vi "FlatToRichniswitch_grpc_InitRequest.vi"(5 "OutputClusterType":T1, 11 "InputCluster":T3) -> (3 "OutputCluster":T1)   [LabVIEW 2021, in "NI Switch_client.lvlib"]
uses:
  NI Switch_client.lvlib
  niswitch_grpc_InitRequest_Flat.ctl
  nidevice_grpc_SessionInitializationBehavior.ctl
  niswitch_grpc_InitRequest.ctl
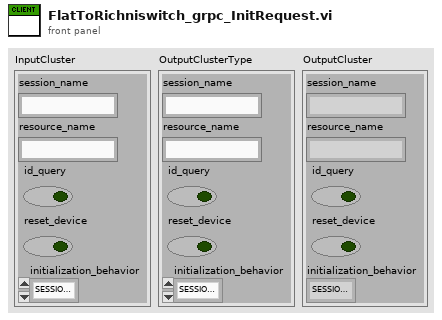
[diagram p1: front panel]
types:
  T1 = typedef "NI Switch_client.lvlib/niswitch_grpc_InitRequest.ctl" = cluster{"session_name":string, "resource_name":string, "id_query":bool, "reset_device":bool, "initialization_behavior":T2}
  T2 = typedef "NI Switch_client.lvlib/nidevice_grpc_SessionInitializationBehavior.ctl" = enum32{"SESSION_INITIALIZATION_BEHAVIOR_UNSPECIFIED", "SESSION_INITIALIZATION_BEHAVIOR_INITIALIZE_NEW", "SESSION_INITIALIZATION_BEHAVIOR_ATTACH_TO_EXISTING"}
  T3 = typedef "NI Switch_client.lvlib/niswitch_grpc_InitRequest_Flat.ctl" = cluster{"session_name":string, "resource_name":string, "id_query":bool, "reset_device":bool, "initialization_behavior":T2}
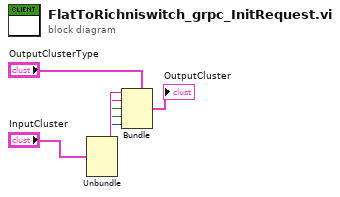
[diagram p0: block diagram]
diagram:
  n1 = Unbundle "Unbundle"("InputCluster") -> ("session_name"=w5:string, "resource_name"=w4:string, "id_query"=w3:bool, "reset_device"=w2:bool, "initialization_behavior"=w1:T2)
  n2 = Bundle "Bundle"(cluster="OutputClusterType", "session_name"=w5, "resource_name"=w4, "id_query"=w3, "reset_device"=w2, "initialization_behavior"=w1) -> (→"OutputCluster":T1)
